vi "unpack_raw.vi"(3 "error in":errorcluster, 5 "u":u64) -> (0 "error out":errorcluster, 1 "raw":string, 2 "u out":u64)   [LabVIEW 2019, in "msgunpack.lvlib"]
doc: "Unpacks a raw byte array from the buffer. Because labview strings can handle the null character, the data is copied and returned as a simple string."
uses:
  msgunpack.lvlib
  msgpack.lvlib
  msgpackalt.dll
panel:
  # "msgpack"
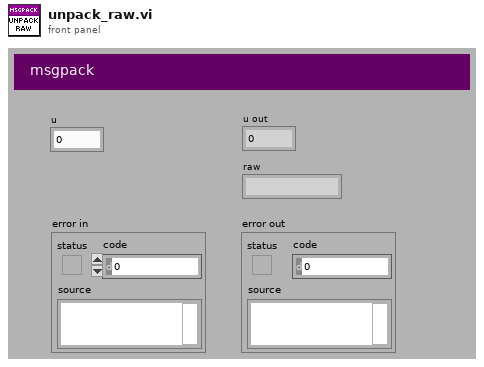
[diagram p1: front panel]
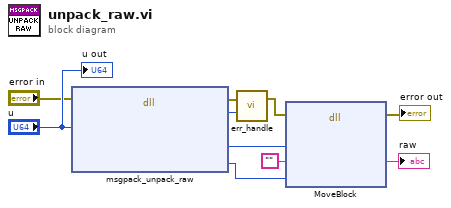
[diagram p0: block diagram]
diagram:
  n1 = dll-call lib="C:/Users/Patrick/Documents/GitHub/Instrument-Framework/lvsrc/SMOs/JSON-RPC-2019/lv-venv/lv.lib/vi.lib/addons/msgpack/msgpackalt.dll" fn="msgpack_unpack_raw"(error in="error in", "p"="u") -> (error out=w7:errorcluster, "return type"=w8:i32, "ptr"=w6:u64, "len"=w5:u32)  [unwired: 5 in, 1 out]
  n2 = call "err_handle.vi"("retval"=w8, "error in"=w7) -> ("error out"=w4:errorcluster)  [unwired: 1 in]
  n3 = dll-call lib="LabVIEW" fn="MoveBlock"(error in=w4, "src"=w6, "dest"="", "len"=w5) -> (error out=→"error out":errorcluster, "dest"=→"raw":string)  [unwired: 5 in, 1 out]
  "u out" <- "u"
